vi "Main.vi"() -> ()   [LabVIEW 2017, in "My Cloneable Module.lvlib"]
doc: "This template is based from the Queued Message Handler design pattern and the Queued Message Handler Project Template that ships with LabVIEW 2014.\n\nThe main difference is that the Queue is private to this module and communication between modules is done via Broadcast and Requests events.\n\nRequests events are wrapped via public API methods and are handled in the Event handler loop in this VI.\nAny module can register for Broadcast events sent by this module.\n\nThe Event Handling Loop generates messages based on user interface actions.\n\nThe Message Handling Loop processes messages generated by the Event Handling Loop, or by other messages. The messages are string values, so new messages can be added easily to the Message Cases case structure in the Message Handling Loop. Each message cluster can also provide an optional value for Message Data, which is a variant that can be converted to whatever message-specific data is required.\n_____\nBased on Delacor QMH Project Template 3.1.0.34."
uses:
  My Cloneable Module.lvlib
  <vilib>/Delacor/Delacor QMH/Libraries/Cloneable Module Admin_class/Delacor_lib_QMH_Cloneable Module Admin.lvclass
  C:/Program Files/National Instruments/LabVIEW 2017/vi.lib/Delacor/Delacor QMH/Libraries/Module Admin_class/Delacor_lib_QMH_Module Admin.lvclass
  Module Data--cluster.ctl
  Do Something Else Argument--cluster.ctl
  Do Something Else and Wait for Reply Argument--cluster.ctl
  Do Something Else and Wait (Reply Payload)--cluster.ctl
  <vilib>/Delacor/Delacor QMH/Libraries/Cloneable Module Admin_class/Delacor_lib_QMH_Cloneable Module Admin.lvclass/Delacor_lib_QMH_Cloneable Module Admin.ctl
  Stop Argument--cluster.ctl
  <vilib>/Delacor/Delacor QMH/Libraries/Module Admin_class/Delacor_lib_QMH_Module Admin.lvclass/Delacor_lib_QMH_Module Admin.ctl
  <vilib>/Utility/miscctls.llb/LVPointTypeDef.ctl
  <vilib>/Delacor/Delacor QMH/Libraries/Cloneable Module Admin_class/Delacor_lib_QMH_Get Module ID.vi
  <vilib>/Delacor/Delacor QMH/Libraries/Module Admin_class/Delacor_lib_QMH_Get External Launch.vi
  <vilib>/Delacor/Delacor QMH/Libraries/Message Queue_class/Delacor_lib_QMH_Enqueue Message (Single).vi
  <vilib>/Utility/error.llb/Error Cluster From Error Code.vi
  <vilib>/ErrorRing/Error Ring.xnode
  <vilib>/Delacor/Delacor QMH/Libraries/Message Queue_class/Delacor_lib_QMH_Message Queue.lvclass
  Clone Registration/Clone Registration.lvlib
panel:
  in  "Simulate MHL Error":bool
  in  "Simulate EHL Error":bool
  out "error out":errorcluster
  in  "Module Admin":refnum<class "Delacor_lib_QMH_Cloneable Module Admin.lvclass">
  out "X":dbl
  out "Status":string
  in  "Do Something Else <Replace Me>":bool
  in  "Do Something <Replace Me>":bool
  # "These controls have associated \"Value Changed\" events configured in the Event Structure on the diagram.\n\nReplace them (and reconfigure the Event Structure) with the controls you need for your application. \n\nOther QMH Modules communicate with this Module via its Public API (wrappers for its Request Events).\n\nThis Module communicates with other Modules via its Broadcast Events.\nAny module that wants to get these messages, just registers for this module's Broadcast events."
  # "This template is for the Delacor Modified Queued Message Handler design pattern.\n\nSee the block diagram for more information on how to use this template."
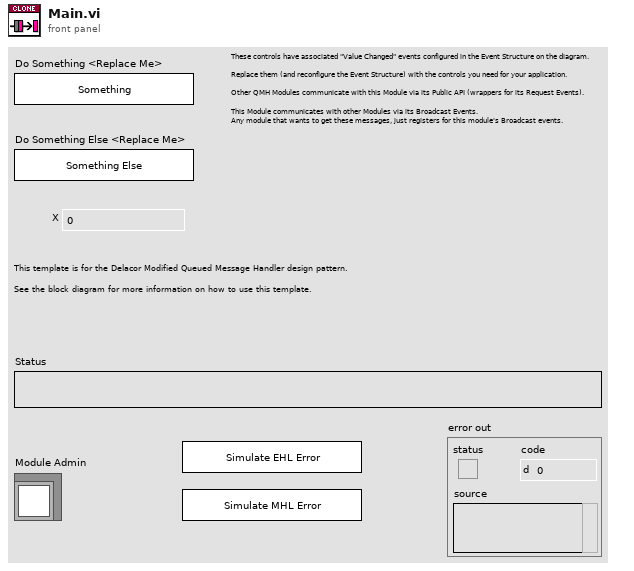
[diagram p1: front panel]
types:
  T1 = typedef "My Cloneable Module.lvlib/Request Events--cluster.ctl" = cluster{"Stop Module":refnum<user-event>, "Do Something":refnum<user-event>, "Do Something Else":refnum<user-event>, "Do Something Else and Wait for Reply":refnum<user-event>, "Show Panel":refnum<user-event>, "Hide Panel":refnum<user-event>, "Show Diagram":refnum<user-event>, "Get Module Execution Status":refnum<user-event>}
  T2 = typedef "My Cloneable Module.lvlib/Module Data--cluster.ctl" = cluster{"Status":string}
  T3 = typedef "My Cloneable Module.lvlib/Do Something Else Argument--cluster.ctl" = cluster{"Do Something Else Msg":string, "X":dbl, "Module ID":i32}
  T4 = typedef "My Cloneable Module.lvlib/Do Something Else and Wait for Reply Argument--cluster.ctl" = cluster{"Do Something Else Msg":string, "X":dbl, "Wait Notifier":refnum<notifier>, "Module ID":i32}
  T5 = typedef "My Cloneable Module.lvlib/Stop Argument--cluster.ctl" = cluster{"Origin":string, "Module ID":i32, "Exit via Stop Module Req?":bool, "Wait for Module to stop?":bool}
  T6 = typedef "LVPointTypeDef.ctl" = cluster{"Horizontal":i16, "Vertical":i16}
  T7 = enum32{"Invalid", "Standard", "Closed", "Hidden", "Minimized", "Maximized"}
  T8 = enum32{"invalid lock state", "Not Locked", "Locked (No Password)", "Password-protected"}
  T9 = typedef "My Cloneable Module.lvlib/Do Something Else and Wait (Reply Payload)--cluster.ctl" = cluster{"Value":dbl, "error":errorcluster}
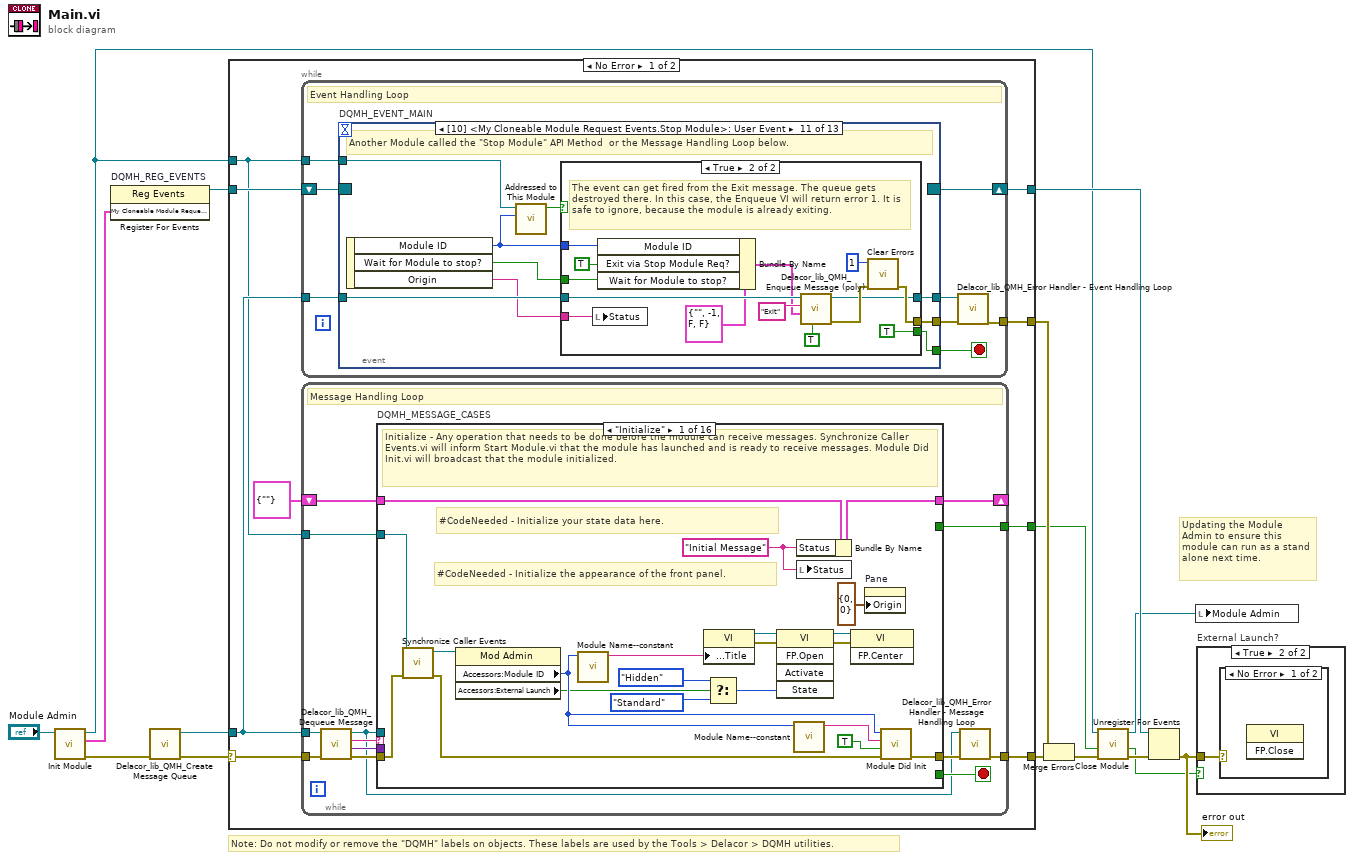
[diagram p0: block diagram]
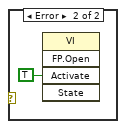
[diagram p3: hidden frame]
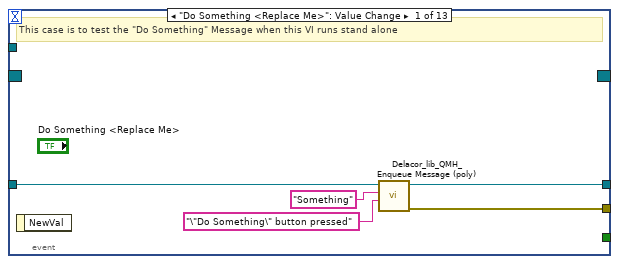
[diagram p4: hidden frame]
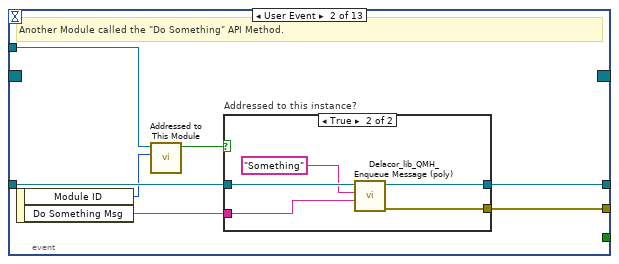
[diagram p5: hidden frame]
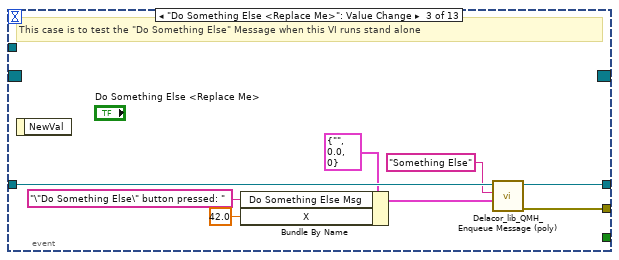
[diagram p7: hidden frame]
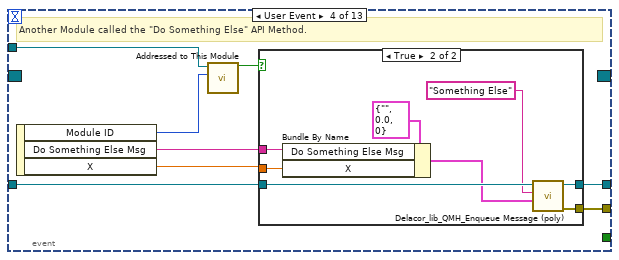
[diagram p8: hidden frame]
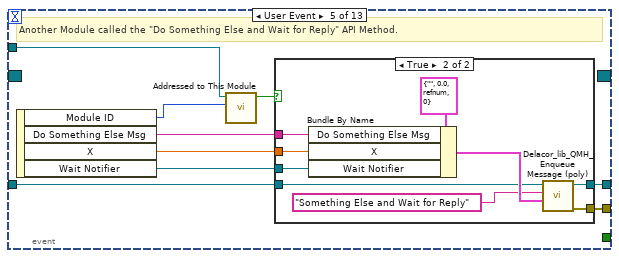
[diagram p10: hidden frame]
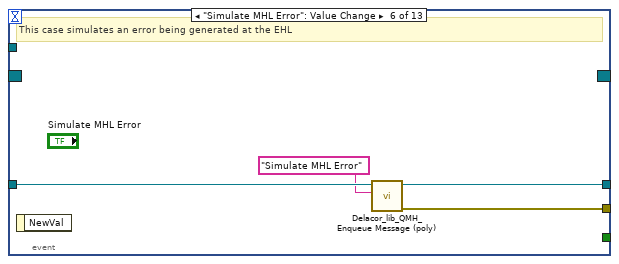
[diagram p12: hidden frame]
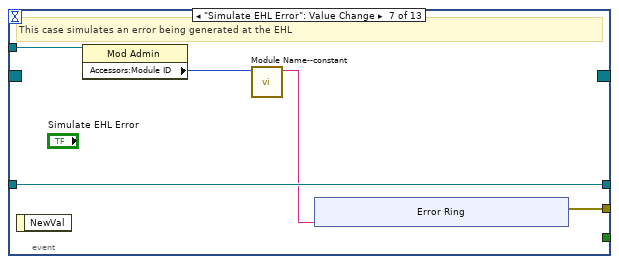
[diagram p13: hidden frame]
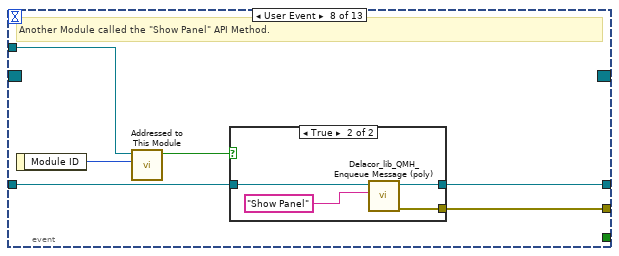
[diagram p14: hidden frame]
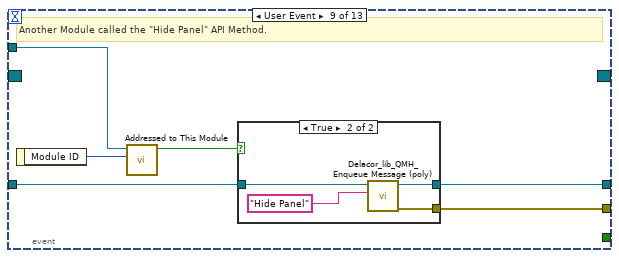
[diagram p16: hidden frame]
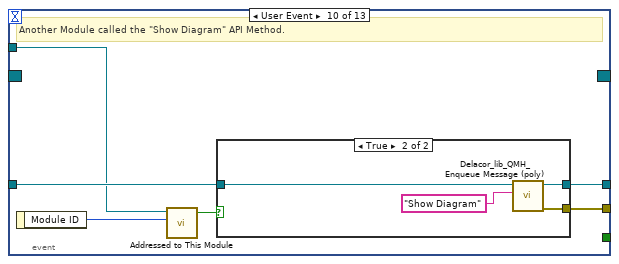
[diagram p18: hidden frame]
diagram:
  # "Note: Do not modify or remove the \"DQMH\" labels on objects. These labels are used by the Tools > Delacor > DQMH utilities."
  # "Updating the Module Admin to ensure this module can run as a stand alone next time."
  n1 = call "Init Module.vi"("Cloneable Module Admin in"="Module Admin") -> ("error out"=w13:errorcluster, "My Cloneable Module Request Events"=w10:T1, "Cloneable Module Admin out"=w6:refnum<class "Delacor_lib_QMH_Cloneable Module Admin.lvclass">)  [unwired: 8 in]
  n2 = register-events "DQMH_REG_EVENTS"(w10) -> (reference out=w11:refnum<event-registration>)  [unwired: 2 in, 1 out]
  n3 = call <vilib>:"Delacor_lib_QMH_Create Message Queue.vi"("error in (no error)"=w13) -> ("error out"=w1:errorcluster, "Message Queue out"=w9:refnum<class "Delacor_lib_QMH_Message Queue.lvclass">)  [unwired: 9 in]
  n4 = case shown="No Error" w1 {
    selector: w1 -> [w19 w401]
    tunnel: [w25 w401] -> w14
    tunnel: [w24 w402] -> w12
    tunnel: w11 -> [w22 w402]
    tunnel: w9 -> [w21 _]
    tunnel: [w20 _] -> w15
    tunnel: w6 -> [w18 w397]
    tunnel: [w17 _] -> w4
    frame No Error {
      n5 = while {
        tunnel: w21 -> [w33]
        shift-right: [w31] -> w24
        shift-left: w22 -> [w32]
        tunnel: [w27] -> w20
        tunnel: w18 -> [w26]
        stop <- w29 stop-if-true
        # "Event Handling Loop"
        n6 = event "DQMH_EVENT_MAIN" shown="[10] <My Cloneable Module Request Events.Stop Module>: User Event" {
          selector: w32 -> [_ _ _ _ _ _ _ _ _ _ _ _ _]
          dyn-events: [_ _ _ _ _ _ _ _ _ _ _ _ _] -> w31
          timeout: _ -> [_ _ _ _ _ _ _ _ _ _ _ _ _]
          tunnel: [_ _ _ _ _ _ _ _ _ _ w148 _ _] -> w29
          tunnel: w33 -> [w38 w45 w59 w67 w80 w99 w104 w117 w128 w139 w151 w176 w180]
          tunnel: [w35 w43 w56 w65 w84 w97 w103 w115 w126 w135 w153 w175 w179] -> w30
          tunnel: [w37 w44 w58 w66 w85 w98 w104 w116 w127 w138 w152 w174 w180] -> w28
          tunnel: w26 -> [_ w39 _ w60 w77 _ w102 w112 w123 w136 w150 w170 w181]
          event "Do Something <Replace Me>": Value Change {
            # "This case is to test the \"Do Something\" Message when this VI runs stand alone"
            n7 = event-data() -> ()  [unwired: 1 in, 1 out]
            n8 = call-poly <vilib>:"Delacor_lib_QMH_Enqueue Message (poly).vi"("Message Data"="\"Do Something\" button pressed" ("\"Do Something\" button pressed"), "Message"="Something", "Message Queue in"=w38) -> ("error out"=w35:errorcluster, "Message Queue out"=w37:refnum<class "Delacor_lib_QMH_Message Queue.lvclass">)  [unwired: 7 in]
          }
          event User Event {
            # "Another Module called the \"Do Something\" API Method."
            n9 = event-data() -> ("Module ID"=w42:i32, "Do Something Msg"=w40:string)  [unwired: 1 in]
            n10 = call "Addressed to This Module.vi"("Module ID from Argument"=w42, "Module Admin"=w39) -> ("Addressed to this instance?"=w41:bool)  [unwired: 8 in, 1 out]
            n11 = case "Addressed to this instance?" shown="True" w41 {
              tunnel: w45 -> [w46 w51]
              tunnel: [w46 w50] -> w44
              tunnel: [_ w48] -> w43
              tunnel: w40 -> [_ w47]
              frame False {
                # "Do nothing"
              }
              frame True {
                n12 = call-poly <vilib>:"Delacor_lib_QMH_Enqueue Message (poly).vi"("Message Data"=w47, "Message"="Something", "Message Queue in"=w51) -> ("error out"=w48:errorcluster, "Message Queue out"=w50:refnum<class "Delacor_lib_QMH_Message Queue.lvclass">)  [unwired: 7 in]
              }
            }
          }
          event "Do Something Else <Replace Me>": Value Change {
            # "This case is to test the \"Do Something Else\" Message when this VI runs stand alone"
            n13 = event-data() -> ()  [unwired: 1 in, 1 out]
            n14 = Bundle By Name(cluster=T3 {"Do Something Else Msg"="", "X"=0.0, "Module ID"=0} ("Do Something Else Argument"), "Do Something Else Msg"="\"Do Something Else\" button pressed: " ("\"Do Something Else\" button pressed"), "X"=42.0) -> (w54:T3)
            n15 = call-poly <vilib>:"Delacor_lib_QMH_Enqueue Message (poly).vi"("Message Data"=w54, "Message"="Something Else", "Message Queue in"=w59) -> ("error out"=w56:errorcluster, "Message Queue out"=w58:refnum<class "Delacor_lib_QMH_Message Queue.lvclass">)  [unwired: 7 in]
          }
          event User Event {
            # "Another Module called the \"Do Something Else\" API Method."
            n16 = event-data() -> ("Module ID"=w61:i32, "Do Something Else Msg"=w64:string, "X"=w63:dbl)  [unwired: 1 in]
            n17 = call "Addressed to This Module.vi"("Module ID from Argument"=w61, "Module Admin"=w60) -> ("Addressed to this instance?"=w62:bool)  [unwired: 8 in, 1 out]
            n18 = case shown="True" w62 {
              tunnel: w67 -> [w68 w76]
              tunnel: [w68 w75] -> w66
              tunnel: [_ w73] -> w65
              tunnel: w64 -> [_ w70]
              tunnel: w63 -> [_ w69]
              frame False {
              }
              frame True {
                n19 = Bundle By Name(cluster=T3 {"Do Something Else Msg"="", "X"=0.0, "Module ID"=0} ("Do Something Else Argument"), "Do Something Else Msg"=w70, "X"=w69) -> (w71:T3)
                n20 = call-poly <vilib>:"Delacor_lib_QMH_Enqueue Message (poly).vi"("Message Data"=w71, "Message"="Something Else", "Message Queue in"=w76) -> ("error out"=w73:errorcluster, "Message Queue out"=w75:refnum<class "Delacor_lib_QMH_Message Queue.lvclass">)  [unwired: 7 in]
              }
            }
          }
          event User Event {
            # "Another Module called the \"Do Something Else and Wait for Reply\" API Method."
            n21 = event-data() -> ("Module ID"=w78:i32, "Do Something Else Msg"=w83:string, "X"=w82:dbl, "Wait Notifier"=w81:refnum<notifier>)  [unwired: 1 in]
            n22 = call "Addressed to This Module.vi"("Module ID from Argument"=w78, "Module Admin"=w77) -> ("Addressed to this instance?"=w79:bool)  [unwired: 8 in, 1 out]
            n23 = case shown="True" w79 {
              tunnel: [w86 w95] -> w85
              tunnel: [_ w94] -> w84
              tunnel: w83 -> [_ w91]
              tunnel: w82 -> [_ w90]
              tunnel: w81 -> [_ w89]
              tunnel: w80 -> [w86 w88]
              frame False {
              }
              frame True {
                n24 = Bundle By Name(cluster=T4 {"Do Something Else Msg"="", "X"=0.0, "Wait Notifier"=refnum, "Module ID"=0} ("Do Something Else and Wait for Reply Argument"), "Do Something Else Msg"=w91, "X"=w90, "Wait Notifier"=w89) -> (w92:T4)
                n25 = call-poly <vilib>:"Delacor_lib_QMH_Enqueue Message (poly).vi"("Message Data"=w92, "Message"="Something Else and Wait for Reply", "Message Queue in"=w88) -> ("error out"=w94:errorcluster, "Message Queue out"=w95:refnum<class "Delacor_lib_QMH_Message Queue.lvclass">)  [unwired: 7 in]
              }
            }
          }
          event "Simulate MHL Error": Value Change {
            # "This case simulates an error being generated at the EHL"
            n26 = event-data() -> ()  [unwired: 1 in, 1 out]
            n27 = call-poly <vilib>:"Delacor_lib_QMH_Enqueue Message (poly).vi"("Message"="Simulate MHL Error", "Message Queue in"=w99) -> ("error out"=w97:errorcluster, "Message Queue out"=w98:refnum<class "Delacor_lib_QMH_Message Queue.lvclass">)  [unwired: 8 in]
          }
          event "Simulate EHL Error": Value Change {
            # "This case simulates an error being generated at the EHL"
            n28 = event-data() -> ()  [unwired: 1 in, 1 out]
            n29 = property class="Mod Admin"(reference=w102) -> ("Accessors:Module ID"=w101:i32)  [unwired: 1 in, 2 out]
            n30 = call "Module Name--constant.vi"("Module ID"=w101) -> ("Module Name"=w100:string)  [unwired: 10 in]
            n31 = xnode "Error Ring"("parameter 0"=w100) -> ("error out"=w103:errorcluster)
          }
          event User Event {
            # "Another Module called the \"Show Panel\" API Method."
            n32 = event-data() -> ("Module ID"=w114:i32)  [unwired: 1 in]
            n33 = call "Addressed to This Module.vi"("Module ID from Argument"=w114, "Module Admin"=w112) -> ("Addressed to this instance?"=w113:bool)  [unwired: 8 in, 1 out]
            n34 = case shown="True" w113 {
              tunnel: w117 -> [w118 w122]
              tunnel: [w118 w121] -> w116
              tunnel: [_ w120] -> w115
              frame False {
              }
              frame True {
                n35 = call-poly <vilib>:"Delacor_lib_QMH_Enqueue Message (poly).vi"("Message"="Show Panel", "Message Queue in"=w122) -> ("error out"=w120:errorcluster, "Message Queue out"=w121:refnum<class "Delacor_lib_QMH_Message Queue.lvclass">)  [unwired: 8 in]
              }
            }
          }
          event User Event {
            # "Another Module called the \"Hide Panel\" API Method."
            n36 = event-data() -> ("Module ID"=w125:i32)  [unwired: 1 in]
            n37 = call "Addressed to This Module.vi"("Module ID from Argument"=w125, "Module Admin"=w123) -> ("Addressed to this instance?"=w124:bool)  [unwired: 8 in, 1 out]
            n38 = case shown="True" w124 {
              tunnel: w128 -> [w129 w133]
              tunnel: [w129 w132] -> w127
              tunnel: [_ w131] -> w126
              frame False {
              }
              frame True {
                n39 = call-poly <vilib>:"Delacor_lib_QMH_Enqueue Message (poly).vi"("Message"="Hide Panel", "Message Queue in"=w133) -> ("error out"=w131:errorcluster, "Message Queue out"=w132:refnum<class "Delacor_lib_QMH_Message Queue.lvclass">)  [unwired: 8 in]
              }
            }
          }
          event User Event {
            # "Another Module called the \"Show Diagram\" API Method."
            n40 = event-data() -> ("Module ID"=w134:i32)  [unwired: 1 in]
            n41 = call "Addressed to This Module.vi"("Module ID from Argument"=w134, "Module Admin"=w136) -> ("Addressed to this instance?"=w137:bool)  [unwired: 8 in, 1 out]
            n42 = case shown="True" w137 {
              tunnel: w139 -> [w140 w144]
              tunnel: [w140 w143] -> w138
              tunnel: [_ w141] -> w135
              frame False {
              }
              frame True {
                n43 = call-poly <vilib>:"Delacor_lib_QMH_Enqueue Message (poly).vi"("Message"="Show Diagram", "Message Queue in"=w144) -> ("error out"=w141:errorcluster, "Message Queue out"=w143:refnum<class "Delacor_lib_QMH_Message Queue.lvclass">)  [unwired: 8 in]
              }
            }
          }
          event User Event {
            # "Another Module called the \"Stop Module\" API Method  or the Message Handling Loop below."
            n44 = event-data() -> ("Module ID"=w146:i32, "Wait for Module to stop?"=w147:bool, "Origin"=w145:string)  [unwired: 1 in]
            n45 = call "Addressed to This Module.vi"("Module ID from Argument"=w146, "Module Admin"=w150) -> ("Addressed to this instance?"=w149:bool)  [unwired: 8 in, 1 out]
            n46 = case shown="True" w149 {
              tunnel: [_ w164] -> w153
              tunnel: [w154 w163] -> w152
              tunnel: w151 -> [w154 w162]
              tunnel: [_ TRUE] -> w148
              tunnel: w147 -> [_ w157]
              tunnel: w146 -> [_ w159]
              tunnel: w145 -> [_ w155]
              frame False {
              }
              frame True {
                # "The event can get fired from the Exit message. The queue gets destroyed there. In this case, the Enqueue VI will return error 1. It is safe to ignore, because the module is already exiting."
                n47 = local write "Status"(w155) -> ()
                n48 = Bundle By Name(cluster=T5 {"Origin"="", "Module ID"=-1, "Exit via Stop Module Req?"=FALSE, "Wait for Module to stop?"=FALSE} ("Stop Argument"), "Module ID"=w159, "Exit via Stop Module Req?"=TRUE, "Wait for Module to stop?"=w157) -> (w156:T5)
                n49 = call-poly <vilib>:"Delacor_lib_QMH_Enqueue Message (poly).vi"("Priority Message? (F)"=TRUE, "Message Data"=w156, "Message"="Exit", "Message Queue in"=w162) -> ("error out"=w167:errorcluster, "Message Queue out"=w163:refnum<class "Delacor_lib_QMH_Message Queue.lvclass">)  [unwired: 6 in]
                n50 = call <vilib>:"Clear Errors.vi"("error in (no error)"=w167, "specific error code to clear (0: all)"=1) -> ("error out"=w164:errorcluster)  [unwired: 4 in, 1 out]
              }
            }
          }
          event Panel Close? {
            w177 = TRUE  # Discard the event so the 'Confirm Quit' message has a chance to run.
            # "If launched externally, closing the panel doesn't quit the VI."
            # "Send the 'Confirm Quit' message if the user closes the panel of the VI."
            n51 = event-data() -> ()  [unwired: 1 in, 1 out]
            n52 = property class="Mod Admin"(reference=w170) -> ("Accessors:External Launch"=w169:bool)  [unwired: 1 in, 2 out]
            n53 = Select(t="Hide Panel" ("Message"), s=w169, f="Confirm Quit" ("Message")) -> (s? t:f=w171:string)
            n54 = call-poly <vilib>:"Delacor_lib_QMH_Enqueue Message (poly).vi"("Message"=w171, "Message Queue in"=w176) -> ("error out"=w175:errorcluster, "Message Queue out"=w174:refnum<class "Delacor_lib_QMH_Message Queue.lvclass">)  [unwired: 8 in]
            n55 = event-data("Discard?"=w177) -> ()  [unwired: 1 in, 1 out]
          }
          event User Event {
            # "For cloneable running as singleton, broadcast that the module is running."
            n56 = event-data() -> ("Module ID"=w178:i32)  [unwired: 1 in]
            n57 = call "Addressed to This Module.vi"("Module ID from Argument"=w178, "Module Admin"=w181) -> ("Addressed to this instance?"=w182:bool)  [unwired: 8 in, 1 out]
            n58 = case shown="True" w182 {
              tunnel: [_ w185] -> w179
              tunnel: w178 -> [_ w184]
              frame False {
              }
              frame True {
                n59 = call "Update Module Execution Status.vi"("Running?"=TRUE, "Module ID"=w184) -> ("error out"=w185:errorcluster)  [unwired: 9 in]
              }
            }
          }
        }
        n60 = call-dynamic "Delacor_lib_QMH_Error Handler - Event Handling Loop.vi"("error in (no error)"=w30, "Message Queue in"=w28) -> ("dup error in"=w27:errorcluster)  [unwired: 8 in, 1 out]
      }
      n61 = while {
        tunnel: w21 -> [w190]
        shift-right: [w196] -> _
        shift-left: T2 {"Status"=""} ("Data Cluster") -> [w197]
        tunnel: w19 -> [w194]
        tunnel: [w188] -> w25
        tunnel: w18 -> [w187]
        tunnel: [w186] -> w17
        stop <- w195 stop-if-true
        # "Message Handling Loop"
        n62 = call-dynamic "Delacor_lib_QMH_Dequeue Message.vi"("error in (no error)"=w194, "Message Queue in"=w190) -> ("error out"=w193:errorcluster, "Message Data"=w191:variant, "Message"=w192:string, "Message Queue out"=w189:refnum<class "Delacor_lib_QMH_Message Queue.lvclass">)  [unwired: 6 in]
        n63 = case "DQMH_MESSAGE_CASES" shown="\"Initialize\"" w192 {
          selector: w192 -> [_ _ _ _ _ _ _ _ _ _ _ _ _ _ _ w384]
          tunnel: w189 -> [_ _ _ _ _ _ w273 w288 w310 _ _ w328 _ w361 w378 _]
          tunnel: w193 -> [w211 w227 w235 w241 w244 w265 w278 w286 w308 w323 w326 w337 w350 w360 w380 _]
          tunnel: [w204 w228 w235 w241 w243 w263 w275 w289 w292 w321 w324 w327 w348 w359 w374 w385] -> w198
          tunnel: w197 -> [w210 w229 w234 w240 w245 w264 w276 w290 w312 w322 w325 w336 w349 w364 w377 w386]
          tunnel: [w209 w229 w234 w240 w245 w264 w276 w290 w312 w322 w325 w336 w349 w364 w377 w386] -> w196
          tunnel: [_ _ _ _ _ _ _ _ _ _ _ _ _ _ w376 _] -> w195
          tunnel: w191 -> [_ w226 _ _ _ _ w270 w282 w304 _ _ w335 _ _ w370 _]
          tunnel: w187 -> [w201 w221 w232 w239 w242 _ w267 _ _ _ _ w332 w345 _ w366 w382]
          tunnel: [_ _ _ _ _ _ _ _ _ _ _ _ _ _ w368 _] -> w186
          frame "Initialize" {
            w208 = "Initial Message" ("Initial Message")
            # "#CodeNeeded - Initialize the appearance of the front panel."
            # "#CodeNeeded - Initialize your state data here."
            # "Initialize - Any operation that needs to be done before the module can receive messages. Synchronize Caller Events.vi will inform Start Module.vi that the module has launched and is ready to receive messages. Module Did Init.vi will broadcast that the module initialized."
            n64 = call "Synchronize Caller Events.vi"("error in (no error)"=w211, "Module Admin"=w201) -> ("error out"=w205:errorcluster, "Module Admin out"=w200:refnum<class "Delacor_lib_QMH_Cloneable Module Admin.lvclass">)  [unwired: 8 in]
            n65 = property class="Mod Admin"(reference=w200) -> ("Accessors:Module ID"=w203:i32, "Accessors:External Launch"=w202:bool)  [unwired: 1 in, 2 out]
            n66 = call "Module Name--constant.vi"("Module ID"=w203) -> ("Module Name"=w215:string)  [unwired: 10 in]
            n67 = property class="VI"("Front Panel.Title"=w215) -> (reference out=w218:refnum<vi>, error out=w219:errorcluster)  [unwired: 2 in]
            n68 = Select(t=T7."Hidden" ("State"), s=w202, f=T7."Standard" ("State")) -> (s? t:f=w212:T7)
            n69 = invoke class="VI" method="FP.Open"(reference=w218, error in=w219, "State"=w212) -> (reference out=w217:refnum<vi>, error out=w216:errorcluster)  [unwired: 2 in, 3 out]
            n70 = call "Module Name--constant.vi"("Module ID"=w203) -> ("Module Name"=w206:string)  [unwired: 10 in]
            n71 = Bundle By Name(cluster=w210, "Status"=w208) -> (w209:T2)
            n72 = local write "Status"(w208) -> ()
            n73 = invoke class="VI" method="FP.Center"(reference=w217, error in=w216) -> ()  [unwired: 1 in, 3 out]
            n74 = property on="Pane" class="Pane"("Origin"=T6 {"Horizontal"=0, "Vertical"=0}) -> ()  [unwired: 2 in, 2 out]
            n75 = call "Module Did Init.vi"("error in (no error)"=w205, "Initialized?"=TRUE, "Origin"=w206, "Module ID"=w203) -> ("error out"=w204:errorcluster)  [unwired: 7 in]
          }
          frame "Update Display" {
            # "Broadcast updated status to any VI registered to listen to this module's broadcast events."
            # "Convert the message data to a string to display in the Status indicator."
            # "#CodeRecommended - If you wish to decouple the Message Handling Loop from your user interface, consider creating User Events (like the \"Stop\" event in this VI) to message the Event Handling Loop whenever the user interface needs updating."
            # "Update Display - Update user interface here."
            n76 = Variant To Data(error in=w227, type="", Variant=w226) -> (data=w224:string, error out=w223:errorcluster)
            "Status" <- w224
            n77 = property class="Mod Admin"(reference=w221) -> ("Accessors:Module ID"=w220:i32)  [unwired: 1 in, 2 out]
            n78 = call "Status Updated.vi"("error in (no error)"=w223, "Status"=w224, "Module ID"=w220) -> ("error out"=w222:errorcluster)  [unwired: 8 in]
            n79 = Merge Errors(w222) -> (w228:errorcluster)
          }
          frame "Show Panel" {
            # "Show the panel of this VI, and send a status updated message to let listeners know."
            n80 = property class="Mod Admin"(reference=w232) -> ("Accessors:Module ID"=w231:i32)  [unwired: 1 in, 2 out]
            n81 = call "Status Updated.vi"("Status"="Panel shown." ("format string"), "Module ID"=w231) -> ()  [unwired: 9 in, 1 out]
            n82 = invoke class="VI" method="FP.Open"("Activate"=TRUE ("Activate?")) -> ()  [unwired: 4 in, 5 out]
          }
          frame "Hide Panel" {
            # "Hide the panel of this VI, and send a status updated message to let listeners know."
            n83 = property class="Mod Admin"(reference=w239) -> ("Accessors:Module ID"=w238:i32)  [unwired: 1 in, 2 out]
            n84 = call "Status Updated.vi"("Status"="Panel hidden." ("format string"), "Module ID"=w238) -> ()  [unwired: 9 in, 1 out]
            n85 = invoke class="VI" method="FP.Open"("State"=T7."Hidden") -> ()  [unwired: 4 in, 5 out]
          }
          frame "Show Diagram" {
            # "Show Diagram - Show the block diagram of this VI. Used as a debugging tool. There is a button in the module tester that fires the Show Diagram request, which runs this message. Note that the diagram will not be displayed if it is password-protected and the password is not in the cache."
            n86 = disable-structure shown="RUN_TIME_ENGINE==False" {
              disable-tunnel: [w254 w262] -> w243
              disable-tunnel: w244 -> [w253 w262]
              disable-tunnel: w242 -> [w246 _]
              frame condition #0 (active) {
                # "functionality not available in exe"
                n87 = invoke class="VI" method="Lock State.Get"(error in=w253) -> (error out=w252:errorcluster, "Get Lock State"=w251:T8, "pwd in cache"=w248:bool)  [unwired: 3 in, 1 out]
                n88 = Equal?(x=T8."Password-protected", y=w251) -> (x = y?=w249:bool)
                n89 = Compound Arithmetic op=AND(w249, invert w248) -> (w247:bool)
                n90 = case shown="False" w247 {
                  tunnel: [w259 w261] -> w254
                  tunnel: w252 -> [w258 w261]
                  tunnel: w246 -> [w255 _]
                  frame False {
                    n91 = property class="Mod Admin"(reference=w255) -> ("Accessors:Module ID"=w256:i32)  [unwired: 1 in, 2 out]
                    n92 = property class="VI"(error in=w258, "BDWin.Open"=TRUE ("Block Diagram Window:Open")) -> (error out=w259:errorcluster)  [unwired: 1 in, 1 out]
                    n93 = call "Status Updated.vi"("Status"="Block Diagram shown." ("format string"), "Module ID"=w256) -> ()  [unwired: 9 in, 1 out]
                  }
                  frame True {
                    # "Password-protected VI, and the password is not in the cache. Do not show the diagram."
                  }
                }
              }
              frame condition #1 {
              }
            }
          }
          frame "--- Module Specific ---" {
            # "Separator -- The following cases handle messages specific to this Module."
            n94 = Merge Errors(w265) -> (w263:errorcluster)
          }
          frame "Something" {
            # "Send string to \"Update Display\" message"
            # "#CodeNeeded - Perform whatever actions correspond to the \"Something\" message."
            # "Something - Replace this message with functionality for your own application. Note that this message also fires the round-trip \"Did Something\" broadcast event."
            n95 = Variant To Data(error in=w278, type="", Variant=w270) -> (data=w266:string, error out=w277:errorcluster)
            n96 = property class="Mod Admin"(reference=w267) -> ("Accessors:Module ID"=w268:i32)  [unwired: 1 in, 2 out]
            n97 = call "Did Something.vi"("error in (no error)"=w277, "Did Something Msg"=w266, "Module ID"=w268) -> ("error out"=w269:errorcluster)  [unwired: 8 in]
            n98 = call-poly <vilib>:"Delacor_lib_QMH_Enqueue Message (poly).vi"("error in (no error)"=w277, "Message Data"=w266, "Message"="Update Display", "Message Queue in"=w273) -> ("error out"=w274:errorcluster)  [unwired: 6 in, 1 out]
            n99 = Merge Errors(w269, w274) -> (w275:errorcluster)
          }
          frame "Something Else" {
            # "Send string to \"Update Display\" message"
            # "#CodeNeeded - Perform whatever actions correspond to the \"Something Else\" message."
            # "Something Else - Replace this message with functionality for your own application."
            n100 = Variant To Data(error in=w286, type=T3 {"Do Something Else Msg"="", "X"=0.0, "Module ID"=0} ("Do Something Else Argument"), Variant=w282) -> (data=w283:T3, error out=w285:errorcluster)
            n101 = Unbundle By Name(w283) -> ("Do Something Else Msg"=w281:string, "X"=w279:dbl)
            "X" <- w279
            n102 = Format Into String(initial string=w281, w279) -> (resulting string=w280:string)  [unwired: 2 in, 1 out]
            n103 = call-poly <vilib>:"Delacor_lib_QMH_Enqueue Message (poly).vi"("error in (no error)"=w285, "Message Data"=w280, "Message"="Update Display", "Message Queue in"=w288) -> ("error out"=w289:errorcluster)  [unwired: 6 in, 1 out]
          }
          frame "Something Else and Wait for Reply" {
            w295 = "X(%.2f)+Offset(%.2f)=%.2f"  # status message format string
            # "Send back X with a random offset"
            # "Something Else and Wait for Reply - Replace this message with functionality for your own application. Note that this message must fire a notifier to let callers know it has finished execution, and it returns an error if the 'Value' is negative."
            n104 = Variant To Data(error in=w308, type=T4 {"Do Something Else Msg"="", "X"=0.0, "Wait Notifier"=refnum, "Module ID"=0} ("Do Something Else and Wait for Reply Argument"), Variant=w304) -> (data=w305:T4, error out=w307:errorcluster)
            n105 = Random Number (0-1)() -> (number: 0 to 1=w296:dbl)
            n106 = Unbundle By Name(w305) -> ("Wait Notifier"=w301:refnum<notifier>, "Do Something Else Msg"=w303:string, "X"=w297:dbl)
            n107 = Add(x=w296, y=w297) -> (x+y=w293:dbl)
            n108 = local write "X"(w297) -> ()
            n109 = flat-sequence {
              tunnel: w301 -> [w320]
              tunnel: [w320] -> w300
              frame #0 {
                # "Simulate an operation that requires a wait."
                n110 = Wait (ms)(milliseconds to wait=u32 1000) -> ()  [unwired: 1 out]
              }
            }
            n111 = Less Than 0?(x=w293) -> (x < 0?=w294:bool)
            n112 = case shown="True" w294 {
              tunnel: [_ w313] -> w291
              frame False {
              }
              frame True {
                n113 = xnode "Error Ring"() -> ("error out"=w313:errorcluster)
              }
            }
            n114 = Format Into String(format string=w295, initial string=w303, w297, w296, w293) -> (resulting string=w302:string)  [unwired: 1 in, 1 out]
            n115 = Bundle By Name(cluster=T9 {"Value"=0.0, "error"={"status"=FALSE, "code"=0, "source"=""}} ("notification"), "Value"=w293, "error"=w291) -> (w298:T9)
            n116 = call-poly <vilib>:"Delacor_lib_QMH_Enqueue Message (poly).vi"("error in (no error)"=w307, "Message Data"=w302, "Message"="Update Display", "Message Queue in"=w310) -> ("error out"=w311:errorcluster)  [unwired: 6 in, 1 out]
            n117 = Merge Errors(w291, w311) -> (w292:errorcluster)
            n118 = Send Notification(notification=w298, notifier=w300) -> ()  [unwired: 1 in, 2 out]
          }
          frame "---Copy This Frame---" {
            # "Duplicate this frame when creating new messages.  Change this comment in the duplicated frame to describe this message."
            n119 = Merge Errors(w323) -> (w321:errorcluster)
          }
          frame "--- Exit and Error Handling---" {
            # "Separator - the following cases handle errors and exit messages."
            n120 = Merge Errors(w326) -> (w324:errorcluster)
          }
          frame "Error" {
            # "#CodeRecommended - If you ever change the name of this \"Error\" message, you'll need to update the name in the Check Loop Error.vi as well."
            # "#CodeRecommended - If the module is running in standalone mode (External Launch = FALSE), this code will pop up an error dialog and call the 'Exit' message if an error occurs. Add more fine-grained error handling here."
            # "Error - Check the error message data and respond accordingly. This message is sent by the \"Error Handler\" VIs at the end of each loop in this application."
            n121 = property class="Mod Admin"(reference=w332) -> ("Accessors:External Launch"=w329:bool, "Accessors:Module ID"=w331:i32)  [unwired: 1 in, 2 out]
            n122 = Variant To Data(error in=w337, type=errorcluster {"status"=FALSE, "code"=0, "source"=""} ("error constant"), Variant=w335) -> (data=w338:errorcluster, error out=w333:errorcluster)
            n123 = call "Error Reported.vi"("Error"=w338, "Module ID"=w331) -> ()  [unwired: 9 in, 1 out]
            n124 = case shown="False" w329 {
              tunnel: [w343 _] -> w330
              tunnel: w328 -> [w342 _]
              tunnel: w338 -> [w339 _]
              frame False {
                # "If the module is running standalone, then pop up an error dialog and call the \"Exit\" message."
                n125 = call <vilib>:"Simple Error Handler.vi"("error in (no error)"=w339) -> ()  [unwired: 4 in, 5 out]
                n126 = call-poly <vilib>:"Delacor_lib_QMH_Enqueue Message (poly).vi"("Priority Message? (F)"=TRUE, "Message"="Exit", "Message Queue in"=w342) -> ("error out"=w343:errorcluster)  [unwired: 7 in, 1 out]
              }
              frame True {
                # "If the module was launched externally, calling the Error Reported broadcast VI is the only action performed by the \"Error\" message. The module's caller can then process the error appropriately."
              }
            }
            n127 = Merge Errors(w333, w330) -> (w327:errorcluster)
            n128 = local write "error out"(w327) -> ()
          }
          frame "Simulate MHL Error" {
            # "Simulate an error occurring at the MHL"
            n129 = property class="Mod Admin"(reference=w345) -> ("Accessors:Module ID"=w346:i32)  [unwired: 1 in, 2 out]
            n130 = call "Module Name--constant.vi"("Module ID"=w346) -> ("Module Name"=w344:string)  [unwired: 10 in]
            n131 = xnode "Error Ring"("parameter 0"=w344) -> ("error out"=w347:errorcluster)
            n132 = Merge Errors(w350, w347) -> (w348:errorcluster)
          }
          frame "Confirm Quit" {
            # "#CodeNeeded - If you want to provide an \"Are you sure\" dialog (or some other notification) before the application exits, place that code here. This message is typically sent from a Panel Close? event."
            # "Confirm Quit - Message that can confirm whether or not the user wants to exit this instance."
            n133 = call-poly <vilib>:"Delacor_lib_QMH_Enqueue Message (poly).vi"("Priority Message? (F)"=TRUE, "error in (no error)"=w360, "Message"="Exit", "Message Queue in"=w361) -> ("error out"=w363:errorcluster)  [unwired: 6 in, 1 out]
            n134 = Merge Errors(w363) -> (w359:errorcluster)
          }
          frame "Exit" {
            w372 = 91  # 91: not all Exit messages will have an argument
            w376 = TRUE  # Stop the VI
            # "Release the message queue reference"
            # "#CodeNeeded - Add any required cleanup code here"
            # "Exit - Exit the application."
            n135 = Variant To Data(error in=w380, type=T5 {"Origin"="", "Module ID"=-1, "Exit via Stop Module Req?"=FALSE, "Wait for Module to stop?"=FALSE} ("Stop Argument"), Variant=w370) -> (data=w367:T5, error out=w371:errorcluster)
            n136 = call <vilib>:"Clear Errors.vi"("error in (no error)"=w371, "specific error code to clear (0: all)"=w372) -> ("error out"=w379:errorcluster)  [unwired: 4 in, 1 out]
            n137 = control-ref of="This VI"() -> (w365:refnum<vi>)
            n138 = call-dynamic "Delacor_lib_QMH_Release Message Queue.vi"("error in (no error)"=w379, "Message Queue"=w378) -> ("error out"=w375:errorcluster)  [unwired: 9 in]
            n139 = call "Handle Exit.vi"("Stop Argument"=w367, "Module Admin in"=w366, "VI reference"=w365) -> ("error out"=w373:errorcluster, "Wait for Stop?"=w368:bool)  [unwired: 7 in]
            n140 = Merge Errors(w373, w375) -> (w374:errorcluster)
          }
          frame Default {
            # "'Default' case only runs if there is a message that isn't defined in any of the other cases.  Output a programming error."
            n141 = property class="Mod Admin"(reference=w382) -> ("Accessors:Module ID"=w381:i32)  [unwired: 1 in, 2 out]
            n142 = call "Module Name--constant.vi"("Module ID"=w381) -> ("Module Name"=w383:string)  [unwired: 10 in]
            n143 = xnode "Error Ring"("parameter 0"=w384, "parameter 1"=w383) -> ("error out"=w385:errorcluster)
          }
        }
        n144 = call-dynamic "Delacor_lib_QMH_Error Handler - Message Handling Loop.vi"("error in (no error)"=w198, "Message Queue in"=w189) -> ("dup error in"=w188:errorcluster)  [unwired: 8 in, 1 out]
      }
    }
    frame Error {
      n145 = call "Synchronize Caller Events.vi"("Module Admin"=w397) -> ("Module Admin out"=w396:refnum<class "Delacor_lib_QMH_Cloneable Module Admin.lvclass">)  [unwired: 9 in, 1 out]
      n146 = property class="Mod Admin"(reference=w396) -> ("Accessors:Module ID"=w395:i32)  [unwired: 1 in, 2 out]
      n147 = call "Module Name--constant.vi"("Module ID"=w395) -> ("Module Name"=w400:string)  [unwired: 10 in]
      n148 = call "Remove.vi"("Module ID"=w395) -> ()  [unwired: 9 in, 2 out]
      n149 = Format Into String(format string="An error occurred during initialization. %s is no longer running.", w400) -> (resulting string=w398:string)  [unwired: 2 in, 1 out]
      n150 = call "Error Reported.vi"("Additional Information"=w398, "Error"=w401, "Module ID"=w395) -> ()  [unwired: 8 in, 1 out]
    }
  }
  n151 = Merge Errors(w15, w14) -> (w16:errorcluster)
  n152 = call "Close Module.vi"("error in (no error)"=w16, "Wait for stop?"=w4, "Module Admin in"=w6) -> ("error out"=w8:errorcluster, "External Launch"=w2:bool, "Module Admin out"=w5:refnum<class "Delacor_lib_QMH_Cloneable Module Admin.lvclass">)  [unwired: 6 in]
  n153 = Unregister For Events(event registration refnum=w12, error in=w8) -> (error out=w3:errorcluster)
  "error out" <- w3
  n154 = local write "Module Admin"(w5) -> ()
  n155 = case "External Launch?" shown="True" w2 {
    tunnel: w3 -> [_ w403]
    frame False {
    }
    frame True {
      n156 = case shown="No Error" w403 {
        frame No Error {
          n157 = invoke class="VI" method="FP.Close"() -> ()  [unwired: 3 in, 3 out]
        }
        frame Error {
          n158 = invoke class="VI" method="FP.Open"("Activate"=TRUE ("Activate?")) -> ()  [unwired: 4 in, 5 out]
        }
      }
    }
  }
